vi "限幅子VI.vi"(1 "波形":waveform(dbl)) -> (0 "输出波形":waveform(dbl))   [LabVIEW 2017]
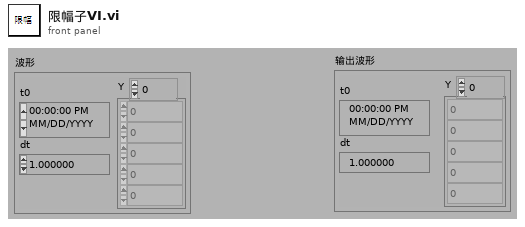
[diagram p1: front panel]
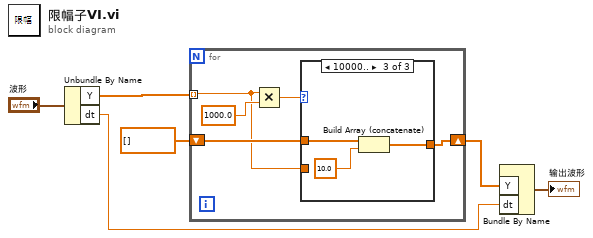
[diagram p0: block diagram]
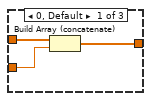
[diagram p2: hidden frame]
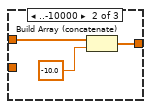
[diagram p3: hidden frame]
diagram:
  n1 = Unbundle By Name("波形") -> ("Y"=w2:dbl[], "dt"=w1:dbl)
  n2 = for {
    tunnel: w2 -> [w8] mode=indexing
    shift-right: [w10] -> w3
    shift-left: dbl[] [] -> [w11]
    n3 = Multiply(x=w8, y=1000.0) -> (x*y=w7:dbl)
    n4 = case shown="10000.." w7 {
      tunnel: w11 -> [w14 w17 w19]
      tunnel: [w12 w16 w18] -> w10
      tunnel: w8 -> [w13 _ _]
      frame 0, Default {
        n5 = Build Array (concatenate)(w14, w13) -> (w12:dbl[])
      }
      frame ..-10000 {
        n6 = Build Array (concatenate)(w17, -10.0 ("y")) -> (w16:dbl[])
      }
      frame 10000.. {
        n7 = Build Array (concatenate)(w19, 10.0 ("y")) -> (w18:dbl[])
      }
    }
  }
  n8 = Bundle By Name("Y"=w3, "dt"=w1) -> (→"输出波形":waveform(dbl))  [unwired: 1 in]
